vi "TraverseControl.vi"(0 "Mode":T1=enum."Read traverse position", 1 "Route Checking?":bool, 3 "Traverse Name":string, 5 "Coordinate rotation (deg)":dbl format="%.2f", 11 "Position input XYZ":dbl[](array[numeric])=[0.0, 0.0, 0.0] format="%.2f", 13 "Speed Factor":dbl=1.0 min=0.1 max=5.0 format="%.2f", 14 "Backlash Compensation?":bool=TRUE) -> (4 "Position Output XYZ":dbl[](array[numeric]) format="%.2f", 15 "Error String":string)   [LabVIEW 2010]
uses:
  Anemometry/Anemometry Sub Vis/Gen Trav/Trav_mode.ctl
  ~subVIs/GenericDriveCommand.ctl
  ADAM Client/Sub VIs/ADAM Controls/Update_scan_value.ctl
  Anemometry/Anemometry Sub Vis/Globals/Trav_pos_global.vi
  Anemometry/Anemometry Sub Vis/Globals/Preference_global.vi
  ~subVIs/DriveConfigGlobal.vi
  Anemometry/Anemometry Sub Vis/Gen Trav/Route mapping/Route_mapping_global.vi
panel:
  out "Server copy Location":path
  out "Position Steps":dbl[][](array[numeric]) format="%.2f"
  out "Log File":path
  out "Achieved Pos In Eng units of all channels":dbl[](array[numeric]) format="%.2f"
  out "Pulses Positon all channels":dbl[](array[numeric])
  out "Counters Reset?":bool
  # "X                Y                   Z"
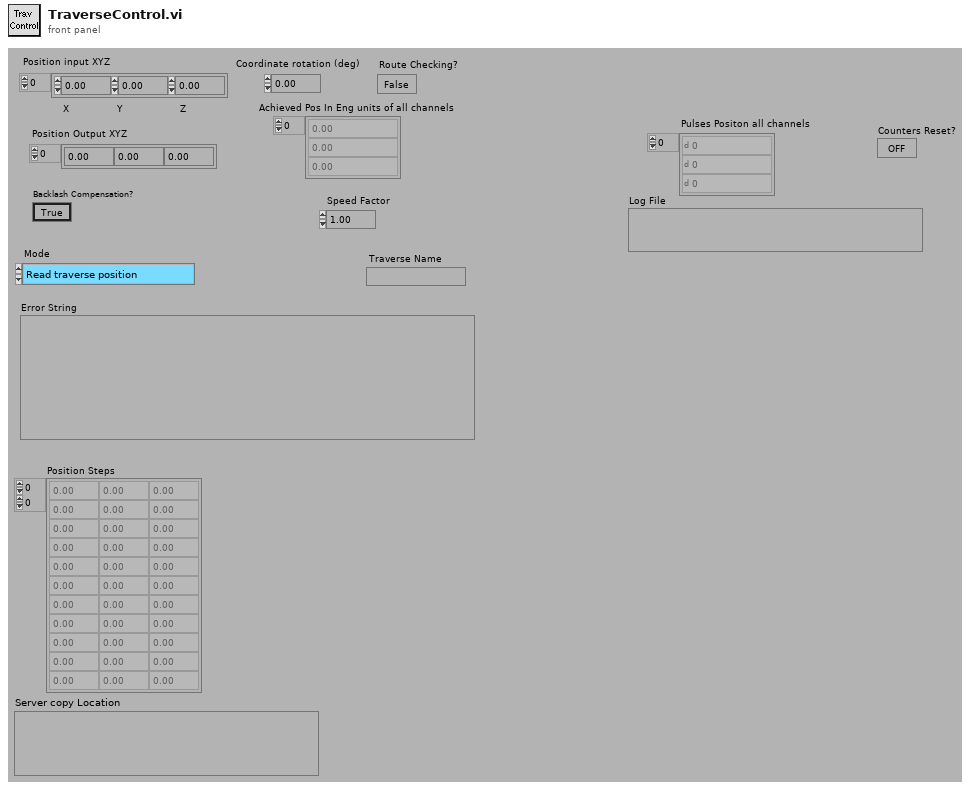
[diagram p1: front panel]
types:
  T1 = typedef "Trav_mode.ctl" = enum16{"Move traverse", "Read traverse position", "Teach Position"}
  T2 = typedef "Tunnel_Coordinates.ctl" = enum16{"Work in Tunnel Coordinates", "Work in Model Coordinates"}
  T3 = typedef "GenericDriveCommand.ctl" = string
  T4 = enum16{"To Traverse Coordinates", "To User Coordinates"}
  T5 = typedef "Update_scan_value.ctl" = cluster{"Channel Name":string, "New Value":dbl}
  T6 = typedef "AxisConfigCluster.ctl" = cluster{"Channel Properties":T7, "Static Drive Configuration":T8}
  T7 = typedef "DriveProperties.ctl" = cluster{"Channel Name":string, "Vel. Default":dbl, "Acc. Default":dbl, "Vel. Max":dbl, "Vel. Min":dbl, "Acc. Max":dbl, "Acc. Min":dbl, "Pulses/unit":dbl, "Address":u8, "Pulse Offset":i32, "Pos Tolerance":dbl, "Pulses/rev":dbl, "Backlash/Eng units":dbl, "Current Pos":dbl, "Ch Status":enum16{"Active", "Offline", "Simulate"}, "Port Name":string, "Axis Transform mode":string, "Metadata Ch Name":string, "Type":string}
  T8 = typedef "DriveStaticConfig.ctl" = cluster{"Correction Gain % (CG)":u16, "Dead Band (DB)":i32, "Dead Band Window (DW)":i32, "Encoder Resolution (ER)":i32, "Step Mode  (FSB)":u16, "Position Maintenance (FSC)":u16, "Stop on Stall (FSD)":u16, "Activate OP1 on stall (FSE)":u16, "Stop on Trigger 3 (FSF)":u16, "OP2 in Deadband (FSG)":u16, "Stall Detect (FSH)":u16, "Limit Disable (LD)":u16, "Motor Resolution (MR)":enum16{"200", "400", "1000", "2000", "4000", "5000", "10000", "12800", "18000", "20000", "21600", "25000", "25400", "25600", "36000", "50000", "278528", "425984", "507904", "614400", "655360", "819200", "1024000"}, "Limit Switch Sense (OSA)":u16, "Home Position (OSB)":u16, "Home Switch Sense (OSC)":u16, "Encoder Z for Home (OSD)":u16, "Reference edge of Home (OSH)":u16, "RS232 Echo Control (SSA)":u16, "Buffer at Limit (SSG)":u16, "Buffer at Stop (SSH)":u16, "Indexer Mode  (FSA)":u16, "Type":string, "ConfigString":string, "De Power Motor":enum16{"TRUE", "FALSE"}}
  T9 = typedef "Box_size.ctl" = cluster{"Max":dbl, "Min":dbl}[]
  T10 = typedef "Exclude_cluster.ctl" = cluster{"Sizes":T9, "Name":string, "Exclude Type":T11}
  T11 = typedef "Exclusion_type.ctl" = enum16{"Exclude completely", "Allow only vertical moves"}
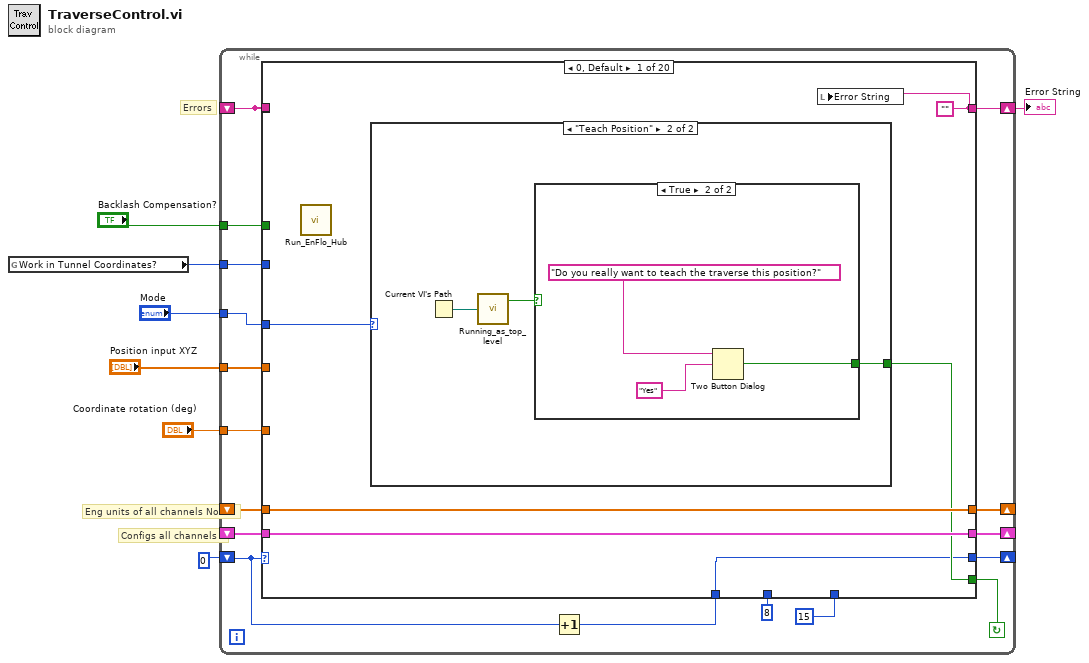
[diagram p0: block diagram]
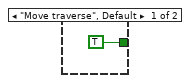
[diagram p2: hidden frame]
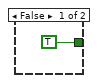
[diagram p3: hidden frame]
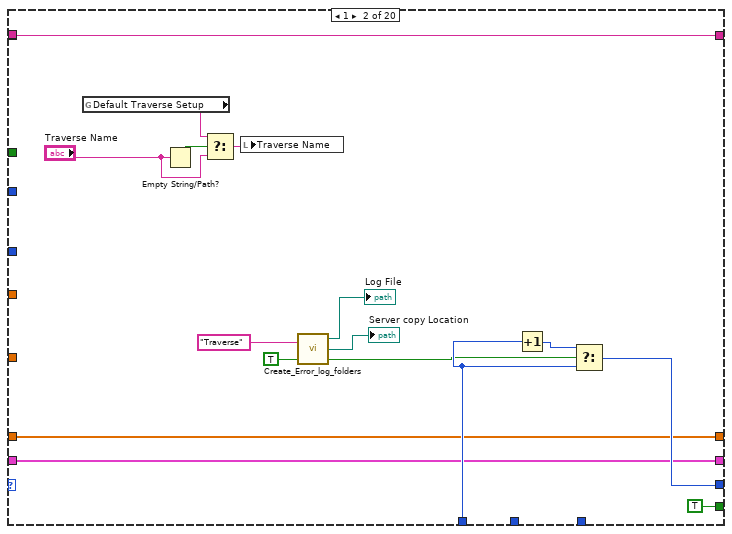
[diagram p4: hidden frame]
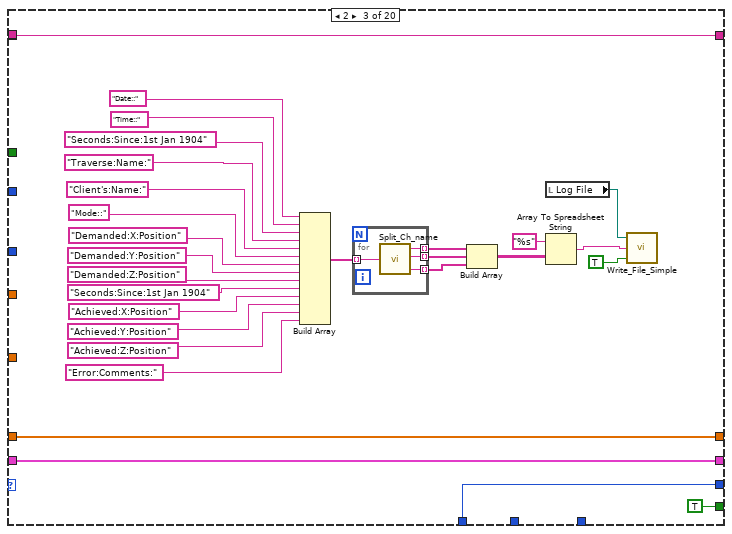
[diagram p5: hidden frame]
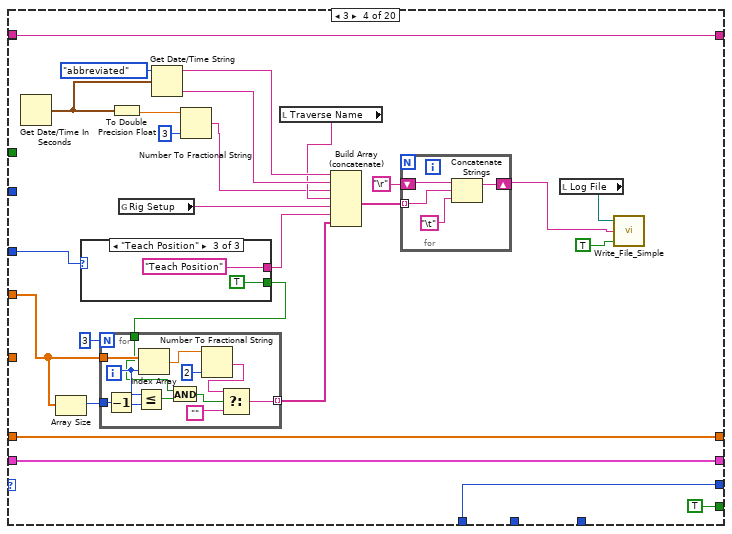
[diagram p6: hidden frame]
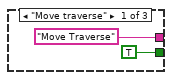
[diagram p7: hidden frame]
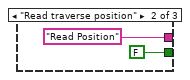
[diagram p8: hidden frame]
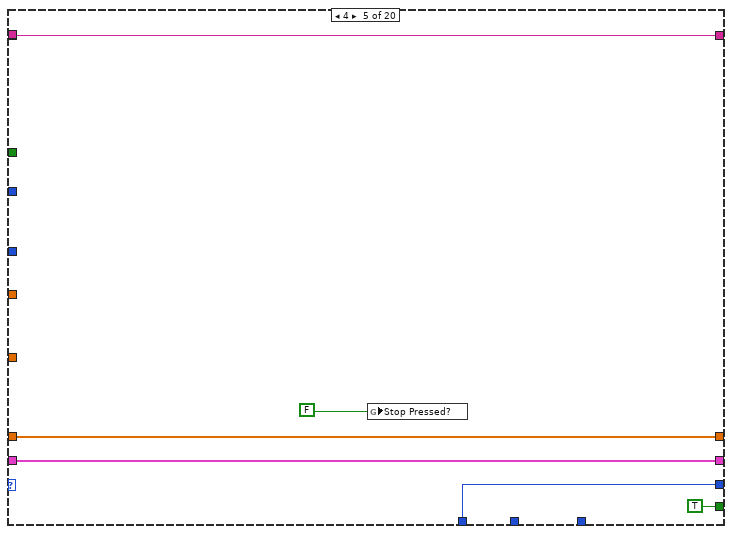
[diagram p9: hidden frame]
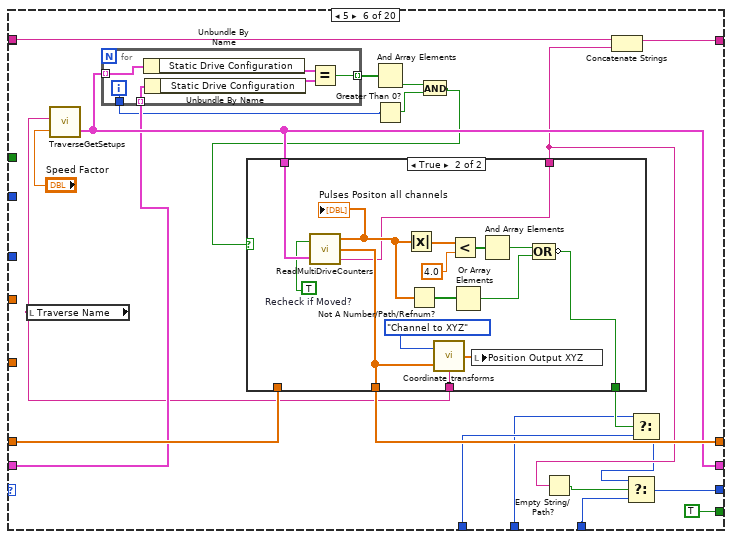
[diagram p10: hidden frame]
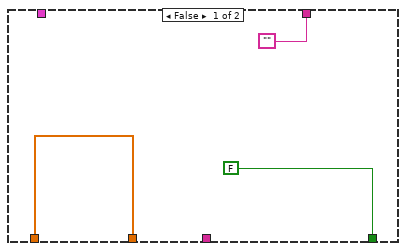
[diagram p11: hidden frame]
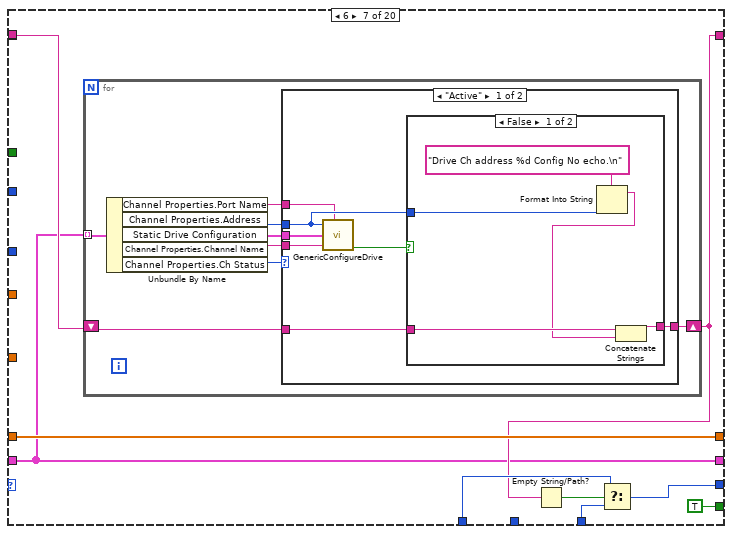
[diagram p12: hidden frame]
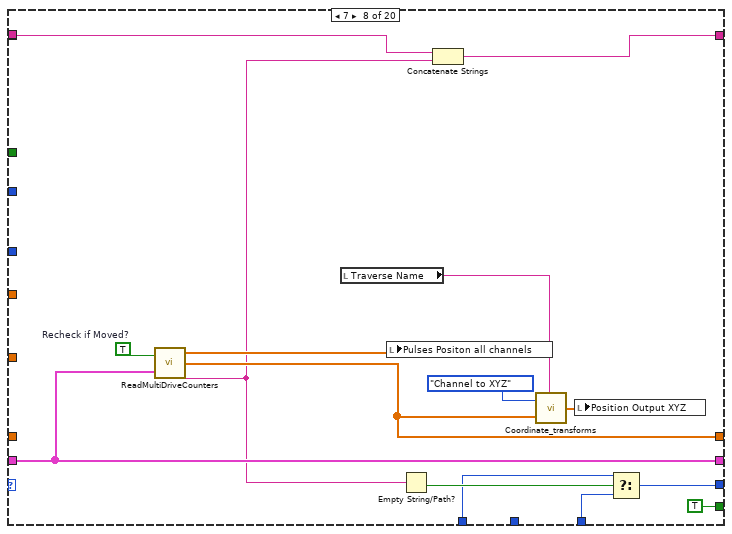
[diagram p15: hidden frame]
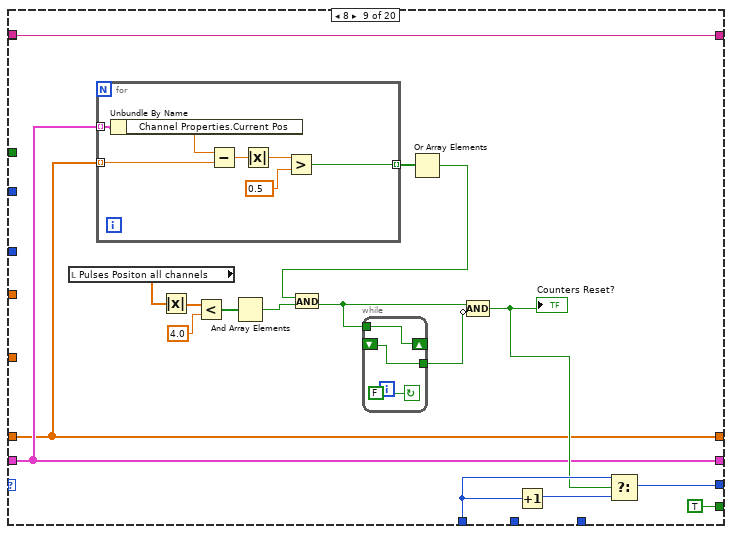
[diagram p16: hidden frame]
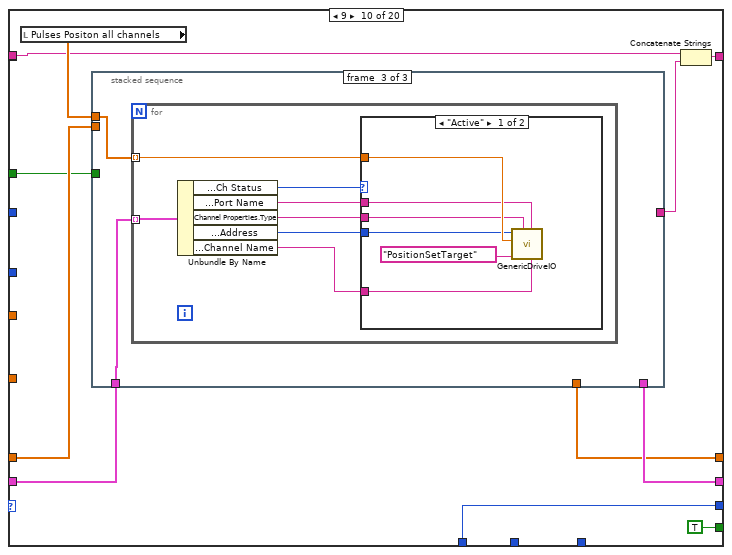
[diagram p17: hidden frame]
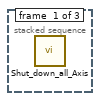
[diagram p18: hidden frame]
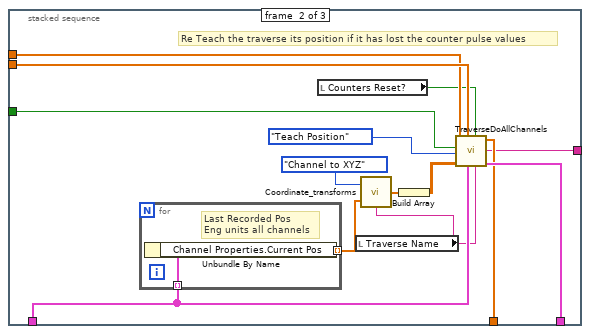
[diagram p19: hidden frame]
diagram:
  # "Errors"
  # "Eng units of all channels Now"
  # "Configs all channels"
  n1 = global read "Trav_pos_global.vi" "Work in Tunnel Coordinates?"() -> (w1:T2)
  n2 = while {
    tunnel: "Backlash Compensation?" -> [w10]
    tunnel: "Position input XYZ" -> [w14]
    shift-left: _ -> [w11]
    shift-right: [w15] -> w5
    shift-left: _ -> [w16]
    shift-right: [w17] -> _
    shift-left: _ -> [w18]
    shift-right: [w19] -> _
    shift-left: 0 -> [w22]
    shift-right: [w20] -> _
    tunnel: "Mode" -> [w24]
    tunnel: "Coordinate rotation (deg)" -> [w9]
    tunnel: w1 -> [w8]
    stop <- w23 continue-if-true
    n3 = Increment(x=w22) -> (x+1=w21:i32)
    n4 = case shown="0, Default" w22 {
      tunnel: w24 -> [w30 _ _ w105 _ _ _ _ _ _ w309 _ w373 w380 _ _ _ w457 _ w513]
      tunnel: [w27 TRUE ("T button?") TRUE ("T button?") TRUE ("T button?") TRUE TRUE ("T button?") TRUE ("T button?") TRUE ("T button?") TRUE TRUE TRUE ("T button?") TRUE ("T button?") TRUE TRUE TRUE ("T button?") TRUE ("T button?") TRUE ("T button?") w459 TRUE FALSE] -> w23
      tunnel: w21 -> [w26 w53 w62 w110 w135 w159 w192 w220 w245 w261 w308 w342 w364 w382 w409 w423 w452 w456 w491 w520]
      tunnel: [w26 w51 w62 w110 w135 w142 w191 w218 w243 w261 w307 w343 w364 w381 w409 w421 w452 w455 w491 w520] -> w20
      tunnel: [w28 w48 w64 w112 w137 w157 w187 w232 w239 w270 w305 w345 w357 w379 w411 w435 w454 w462 w489 w518] -> w19
      tunnel: w18 -> [w28 w48 w64 w112 w137 w156 w187 w232 w239 w269 w305 w345 w371 w379 w411 w435 w454 w462 w489 w518]
      tunnel: [w29 w49 w63 w111 w138 w162 w195 w227 w238 w266 w304 w329 w365 w385 w410 w434 w453 w463 w492 w521] -> w17
      tunnel: w16 -> [w29 w49 w63 w111 w138 w161 w195 _ w238 w267 w304 w329 w360 w385 w410 w434 w453 w463 w492 w521]
      tunnel: [w25 w47 w60 w102 w139 w147 w188 w223 w242 w263 w310 w334 w367 w383 w407 w425 w450 w458 w485 w514] -> w15
      tunnel: w11 -> [_ w47 w60 w102 w139 w148 w189 w224 w242 w265 w310 _ w368 w383 w407 w425 w450 w461 w487 w516]
      tunnel: w14 -> [_ _ _ w99 _ _ _ _ _ _ w303 w331 _ _ _ _ _ _ w483 _]
      tunnel: 15 ("f") -> [_ _ _ _ _ w143 w190 w219 _ _ _ w336 _ _ _ _ _ _ _ _]
      tunnel: 8 ("t") -> [_ _ _ _ _ w158 _ _ _ _ _ _ _ _ _ _ _ _ _ _]
      tunnel: w11 -> [_ _ _ _ _ _ _ _ _ _ _ w337 _ _ _ _ _ _ _ _]
      tunnel: w10 -> [_ _ _ _ _ _ _ _ _ w260 _ _ w359 _ _ _ _ _ _ _]
      tunnel: w9 -> [_ _ _ _ _ _ _ _ _ _ _ w325 _ _ _ _ _ _ w484 w511]
      tunnel: w8 -> [_ _ _ _ _ _ _ _ _ _ _ _ _ _ _ _ _ _ w481 w509]
      frame 0, Default {
        w25 = ""
        n5 = call "Run_EnFlo_Hub.vi"() -> ()  [unwired: 8 out]
        n6 = case shown="\"Teach Position\"" w30 {
          tunnel: [TRUE ("T button?") w32] -> w27
          frame "Move traverse", Default {
          }
          frame "Teach Position" {
            n7 = Current VI's Path() -> (path=w34:path)
            n8 = call "Running_as_top_level.vi"("Vi path name"=w34) -> ("Top Level"=w33:bool)  [unwired: 1 out]
            n9 = case shown="True" w33 {
              tunnel: [TRUE ("T button?") w36] -> w32
              frame False {
              }
              frame True {
                n10 = Two Button Dialog(message="Do you really want to teach the traverse this position?", 2:"Yes" ("T button name (\"OK\")")) -> (T button?=w36:bool)  [unwired: 1 out]
              }
            }
          }
        }
        n11 = local write "Error String"(w25) -> ()
      }
      frame 1 {
        n12 = global read "Trav_pos_global.vi" "Default Traverse Setup"() -> (w44:string)
        n13 = Empty String/Path?(string/path="Traverse Name") -> (empty?=w42:bool)
        n14 = Select(t=w44, s=w42, f="Traverse Name") -> (s? t:f=w41:string)
        n15 = local write "Traverse Name"(w41) -> ()
        n16 = call "Create_Error_log_folders.vi"("Per Day Log File?"=TRUE, "Log Filename"="Traverse" ("Input Element")) -> ("exists?"=w45:bool, "Server copy Location"=→"Server copy Location":path, "Local Log File"=→"Log File":path)  [unwired: 1 in]
        n17 = Increment(x=w53) -> (x+1=w52:i32)
        n18 = Select(t=w52, s=w45, f=w53) -> (s? t:f=w51:i32)
      }
      frame 2 {
        n19 = Build Array("Date::", "Time::", "Seconds:Since:1st Jan 1904", "Traverse:Name:", "Client's:Name:", "Mode::", "Demanded:X:Position", "Demanded:Y:Position", "Demanded:Z:Position", "Seconds:Since:1st Jan 1904", "Achieved:X:Position", "Achieved:Y:Position", "Achieved:Z:Position", "Error:Comments:") -> (w67:string[])
        n20 = for {
          tunnel: w67 -> [w86] mode=indexing
          tunnel: [w85] -> w68 mode=indexing
          tunnel: [w84] -> w69 mode=indexing
          tunnel: [w83] -> w70 mode=indexing
          n21 = call "Split_Ch_name.vi"("Ch name"=w86) -> ("Top level"=w85:string, "Middle"=w84:string, "Low level"=w83:string)
        }
        n22 = Build Array(w68, w69, w70) -> (w65:string[][])
        n23 = local read "Log File"() -> (w56:path)
        n24 = Array To Spreadsheet String(array=w65, 3:"%s" ("format string")) -> (spreadsheet string=w57:string)  [unwired: 1 out]
        n25 = call "Write_File_Simple.vi"("append to file? (new file:F)"=TRUE, "character string"=w57, "file path"=w56) -> ()  [unwired: 2 out]
      }
      frame 3 {
        n26 = Get Date/Time In Seconds() -> (seconds since 1Jan1904=w91:timestamp)
        n27 = Array Size(array=w99) -> (size(s)=w100:i32)
        n28 = case shown="\"Teach Position\"" w105 {
          tunnel: ["Move Traverse" "Read Position" "Teach Position"] -> w106
          tunnel: [TRUE FALSE TRUE] -> w96
          frame "Move traverse" {
          }
          frame "Read traverse position" {
          }
          frame "Teach Position" {
          }
        }
        n29 = for {
          N: 3 -> [_]
          tunnel: w99 -> [w124]
          tunnel: w100 -> [w121]
          tunnel: [w117] -> w97 mode=indexing
          tunnel: w96 -> [w113]
          i -> [w119]
          n30 = Decrement(x=w121) -> (x-1=w120:i32)
          n31 = Less Or Equal?(x=w119, y=w120) -> (x <= y?=w115:bool)
          n32 = Index Array(array=w124, index=w119) -> (element=w123:dbl)
          n33 = And(x=w113, y=w115) -> (x .and. y?=w114:bool)
          n34 = Number To Fractional String(number=w123, precision (6)=i16 2) -> (F-format string=w118:string)  [unwired: 2 out]
          n35 = Select(t=w118, s=w114, f="") -> (s? t:f=w117:string)
        }
        n36 = To Double Precision Float(number=w91) -> (double precision float=w90:dbl)
        n37 = global read "Preference_global.vi" "Rig Setup"() -> (w87:string)
        n38 = Get Date/Time String(date format (0)=enum16{"short", "long", "abbreviated"}."abbreviated", seconds (now)=w91) -> (date string=w108:string, time string=w107:string)  [unwired: 1 out]
        n39 = Number To Fractional String(number=w90, precision (6)=i16 3) -> (F-format string=w88:string)  [unwired: 2 out]
        n40 = local read "Traverse Name"() -> (w92:string)
        n41 = Build Array (concatenate)(w108, w107, w88, w92, w87, w106, w97) -> (w103:string[])
        n42 = for {
          shift-right: [w127] -> w93
          shift-left: "\r" -> [w128]
          tunnel: w103 -> [w126] mode=indexing
          n43 = Concatenate Strings(w128, w126, "\t") -> (w127:string)
        }
        n44 = local read "Log File"() -> (w94:path)
        n45 = call "Write_File_Simple.vi"("append to file? (new file:F)"=TRUE, "character string"=w93, "file path"=w94) -> ()  [unwired: 2 out]
      }
      frame 4 {
        n46 = global write "DriveConfigGlobal.vi" "Stop Pressed?"(FALSE) -> ()
      }
      frame 5 {
        n47 = local read "Traverse Name"() -> (w150:string)
        n48 = call "TraverseGetSetups.vi"("Speed Factor"="Speed Factor", "Traverse Name"=w150) -> ("Matched Configurations"=w157:T6[])  [unwired: 1 out]
        n49 = for {
          tunnel: w157 -> [w168] mode=indexing
          tunnel: w156 -> [w167] mode=indexing
          tunnel: [w164] -> w155 mode=indexing
          tunnel: [w163] -> w154
          i -> [w163]
          n50 = Unbundle By Name(w168) -> ("Static Drive Configuration"=w166:T8)
          n51 = Unbundle By Name(w167) -> ("Static Drive Configuration"=w165:T8)
          n52 = Equal?(x=w166, y=w165) -> (x = y?=w164:bool)
        }
        n53 = And Array Elements(Boolean array=w155) -> (logical AND=w152:bool)
        n54 = Greater Than 0?(x=w154) -> (x > 0?=w153:bool)
        n55 = And(x=w152, y=w153) -> (x .and. y?=w151:bool)
        n56 = case shown="True" w151 {
          tunnel: w157 -> [_ w186]
          tunnel: [w171 w176] -> w162
          tunnel: w161 -> [w171 _]
          tunnel: [FALSE w178] -> w160
          tunnel: w150 -> [_ w174]
          tunnel: ["" w172] -> w146
          frame False {
          }
          frame True {
            w173 = TRUE  # Recheck if Moved?
            n57 = call "ReadMultiDriveCounters.vi"("Recheck if Moved?"=w173, "Matched Configurations"=w186) -> ("Pulses"=w181:dbl[], "Eng units"=w176:dbl[], "Error String"=w172:string)
            "Pulses Positon all channels" <- w181
            n58 = Absolute Value(x=w181) -> (abs(x)=w185:dbl[])
            n59 = Not A Number/Path/Refnum?(number/path/refnum=w181) -> (NaN/Path/Refnum?=w180:bool[])
            n60 = call "Coordinate_transforms.vi"("Traverse Name"=w174, "Input"=w176, "Mode"=enum16{"XYZ to Channel", "Channel to XYZ"}."Channel to XYZ") -> ("Output"=w175:dbl[])
            n61 = Less?(x=w185, y=4.0 ("Achieved Position")) -> (x < y?=w183:bool[])
            n62 = Or Array Elements(Boolean array=w180) -> (logical OR=w179:bool)
            n63 = local write "Position Output XYZ"(w175) -> ()
            n64 = And Array Elements(Boolean array=w183) -> (logical AND=w182:bool)
            n65 = Compound Arithmetic op=OR(w182, w179) -> (invert w178:bool)
          }
        }
        n66 = Empty String/Path?(string/path=w146) -> (empty?=w145:bool)
        n67 = Concatenate Strings(w148, w146) -> (w147:string)
        n68 = Select(t=w158, s=w160, f=w159) -> (s? t:f=w144:i32)
        n69 = Select(t=w144, s=w145, f=w143) -> (s? t:f=w142:i32)
      }
      frame 6 {
        n70 = for {
          tunnel: w187 -> [w203] mode=indexing
          shift-right: [w196] -> w188
          shift-left: w189 -> [w197]
          n71 = Unbundle By Name(w203) -> ("Channel Properties.Port Name"=w198:string, "Channel Properties.Address"=w202:u8, "Static Drive Configuration"=w201:T8, "Channel Properties.Channel Name"=w200:string, "Channel Properties.Ch Status"=w199:enum16{"Active", "Offline", "Simulate"})
          n72 = case shown="\"Active\"" w199 {
            tunnel: w202 -> [w208 _]
            tunnel: w201 -> [w210 _]
            tunnel: w200 -> [w209 _]
            tunnel: w198 -> [w207 _]
            tunnel: w197 -> [w205 w217]
            tunnel: [w204 w217] -> w196
            frame "Active" {
              n73 = call "GenericConfigureDrive.vi"("Address"=w208, "Port Name"=w207, "Static Drive Configuration"=w210, "Channel Name"=w209) -> ("Good Echo"=w206:bool)  [unwired: 4 out]
              n74 = case shown="False" w206 {
                tunnel: w208 -> [w215 _]
                tunnel: w205 -> [w213 w216]
                tunnel: [w212 w216] -> w204
                frame False {
                  n75 = Format Into String(format string="Drive Ch address %d Config No echo.\n" ("Format String"), w215) -> (resulting string=w211:string)  [unwired: 2 in, 1 out]
                  n76 = Concatenate Strings(w213, w211) -> (w212:string)
                }
                frame True {
                }
              }
            }
            frame "Offline", Default {
            }
          }
        }
        n77 = Empty String/Path?(string/path=w188) -> (empty?=w193:bool)
        n78 = Select(t=w192, s=w193, f=w190) -> (s? t:f=w191:i32)
      }
      frame 7 {
        w225 = TRUE  # Recheck if Moved?
        n79 = call "ReadMultiDriveCounters.vi"("Recheck if Moved?"=w225, "Matched Configurations"=w232) -> ("Pulses"=w230:dbl[], "Eng units"=w227:dbl[], "Error String"=w221:string)
        n80 = local read "Traverse Name"() -> (w226:string)
        n81 = local write "Pulses Positon all channels"(w230) -> ()
        n82 = Empty String/Path?(string/path=w221) -> (empty?=w222:bool)
        n83 = Concatenate Strings(w224, w221) -> (w223:string)
        n84 = call "Coordinate_transforms.vi"("Traverse Name"=w226, "Input"=w227, "Mode"=enum16{"XYZ to Channel", "Channel to XYZ"}."Channel to XYZ") -> ("Output"=w228:dbl[])
        n85 = local write "Position Output XYZ"(w228) -> ()
        n86 = Select(t=w220, s=w222, f=w219) -> (s? t:f=w218:i32)
      }
      frame 8 {
        n87 = local read "Pulses Positon all channels"() -> (w233:dbl[])
        n88 = for {
          tunnel: w239 -> [w259] mode=indexing
          tunnel: w238 -> [w257] mode=indexing
          tunnel: [w253] -> w236 mode=indexing
          n89 = Unbundle By Name(w259) -> ("Channel Properties.Current Pos"=w258:dbl)
          n90 = Subtract(x=w258, y=w257) -> (x-y=w256:dbl)
          n91 = Absolute Value(x=w256) -> (abs(x)=w255:dbl)
          n92 = Greater?(x=w255, y=0.5) -> (0:w253:bool)
        }
        n93 = Absolute Value(x=w233) -> (abs(x)=w249:dbl[])
        n94 = Less?(x=w249, y=4.0 ("Achieved Position")) -> (x < y?=w247:bool[])
        n95 = And Array Elements(Boolean array=w247) -> (logical AND=w237:bool)
        n96 = Or Array Elements(Boolean array=w236) -> (logical OR=w235:bool)
        n97 = And(x=w235, y=w237) -> (x .and. y?=w234:bool)
        n98 = while {
          tunnel: [w251] -> w241
          tunnel: w234 -> [w252]
          shift-left: _ -> [w251]
          shift-right: [w252] -> _
          stop <- FALSE continue-if-true
        }
        n99 = Compound Arithmetic op=AND(w234, invert w241) -> (w240:bool)
        "Counters Reset?" <- w240
        n100 = Increment(x=w245) -> (x+1=w244:i32)
        n101 = Select(t=w245, s=w240, f=w244) -> (s? t:f=w243:i32)
      }
      frame 9 {
        n102 = local read "Pulses Positon all channels"() -> (w268:dbl[])
        n103 = stacked-sequence {
          tunnel: w268 -> [_ w276 w287]
          tunnel: [_ w284 _] -> w270
          tunnel: w267 -> [_ w283 _]
          tunnel: [_ w282 _] -> w266
          tunnel: w269 -> [_ w278 w288]
          tunnel: [_ w281 _] -> w264
          tunnel: w260 -> [_ w272 _]
          frame #0 {
            n104 = call "Shut_down_all_Axis.vi"() -> ()  [unwired: 1 out]
          }
          frame #1 {
            # "Re Teach the traverse its position if it has lost the counter pulse values"
            n105 = for {
              tunnel: [w286] -> w277 mode=indexing
              tunnel: w278 -> [w285] mode=indexing
              # "Last Recorded Pos\nEng units all channels"
              n106 = Unbundle By Name(w285) -> ("Channel Properties.Current Pos"=w286:dbl)
            }
            n107 = local read "Counters Reset?"() -> (w274:bool)
            n108 = local read "Traverse Name"() -> (w273:string)
            n109 = call "Coordinate_transforms.vi"("Traverse Name"=w273, "Input"=w277, "Mode"=enum16{"XYZ to Channel", "Channel to XYZ"}."Channel to XYZ") -> ("Output"=w279:dbl[])
            n110 = Build Array(w279) -> (w271:dbl[][])
            n111 = call "TraverseDoAllChannels.vi"("Traverse Name"=w273, "Counters Reset?"=w274, "Matched Configurations all Channels In"=w278, "Current Pos In Eng units of all channels"=w283, "Position Steps"=w271, "Mode"=Trav_mode."Teach Position", "Backlash Compensation?"=w272, "Current Pulses positions for all channels"=w276) -> ("Matched Configurations Out"=w284:T6[], "Error String"=w281:string, "Achieved Pos In Eng units of all channels"=w282:dbl[])  [unwired: 1 out]
          }
          frame #2 {
            n112 = for {
              tunnel: w288 -> [w295] mode=indexing
              tunnel: w287 -> [w294] mode=indexing
              n113 = Unbundle By Name(w295) -> ("Channel Properties.Ch Status"=w293:enum16{"Active", "Offline", "Simulate"}, "Channel Properties.Port Name"=w292:string, "Channel Properties.Type"=w291:string, "Channel Properties.Address"=w290:u8, "Channel Properties.Channel Name"=w289:string)
              n114 = case shown="\"Active\"" w293 {
                tunnel: w294 -> [w301 _]
                tunnel: w292 -> [w300 _]
                tunnel: w291 -> [w299 _]
                tunnel: w290 -> [w298 _]
                tunnel: w289 -> [w297 _]
                frame "Active" {
                  n115 = call "GenericDriveIO.vi"("GenericDriveCommand"=T3 "PositionSetTarget", "Channel Name"=w297, "Numeric Value"=w301, "Address"=w298, "Type"=w299, "Port Name"=w300) -> ()  [unwired: 1 in, 5 out]
                }
                frame "Offline", Default {
                }
              }
            }
          }
        }
        n116 = Concatenate Strings(w265, w264) -> (w263:string)
      }
      frame 10 {
        n117 = Build Array(w303) -> (w302:dbl[][])
        n118 = local write "Position Steps"(w302) -> ()
        n119 = case shown="\"Read traverse position\", Default" w309 {
          tunnel: w308 -> [w311 w318]
          tunnel: [w313 w317] -> w307
          frame "Move traverse" {
            n120 = Increment(x=w311) -> (x+1=w312:i32)
            n121 = case shown="True" "Route Checking?" {
              tunnel: [w315 w316] -> w313
              tunnel: w312 -> [w315 _]
              tunnel: w311 -> [_ w316]
              frame False {
              }
              frame True {
              }
            }
          }
          frame "Read traverse position", Default {
            n122 = Increment(x=w318) -> (x+1=w317:i32)
          }
        }
      }
      frame 11 {
        w321 = 0.1  # Reduce by
        w328 = TRUE  # Full Check
        n123 = global read "Route_mapping_global.vi" "Probe Volume"() -> (w320:T9)
        n124 = local read "Traverse Name"() -> (w330:string)
        n125 = for {
          tunnel: w320 -> [w352] mode=indexing
          tunnel: [w351] -> w319 mode=indexing
          tunnel: w321 -> [w346]
          n126 = Unbundle By Name(w352) -> ("Max"=w350:dbl, "Min"=w348:dbl)
          n127 = Subtract(x=w350, y=w346) -> (x-y=w349:dbl)
          n128 = Add(x=w346, y=w348) -> (x+y=w347:dbl)
          n129 = Bundle By Name(cluster=w352, "Max"=w349, "Min"=w347) -> (w351:cluster{"Max":dbl, "Min":dbl})
        }
        n130 = global read "Route_mapping_global.vi" "Entire Space"() -> (w322:T9)
        n131 = global read "Route_mapping_global.vi" "Exclude Array"() -> (w323:T10[])
        n132 = call "Coordinate_transforms.vi"("Traverse Name"=w330, "Input"=w329, "Mode"=enum16{"XYZ to Channel", "Channel to XYZ"}."Channel to XYZ") -> ("Output"=w332:dbl[])
        n133 = call "Coordinate_rotation.vi"("Input Position"=w332, "Coordinate rotation (deg)"=w325, "Mode"=T4."To User Coordinates") -> ("Output Position"=w339:dbl[])
        n134 = call "Coordinate_rotation.vi"("Input Position"=w331, "Coordinate rotation (deg)"=w325, "Mode"=T4."To User Coordinates") -> ("Output Position"=w338:dbl[])
        n135 = call "Check_Traverse_move.vi"("Current position"=w339, "Traverse Name"=w330, "Full Check"=w328, "New Position"=w338, "Coordinate rotation (deg)"=w325, "Probe Volume"=w319, "Entire Space"=w322, "Exclude Array"=w323) -> ("Steps"=w327:dbl[][], "Error Comments"=w324:string)  [unwired: 6 out]
        n136 = Empty String/Path?(string/path=w324) -> (empty?=w335:bool)
        n137 = for {
          tunnel: w327 -> [w355] mode=indexing
          tunnel: [w354] -> w326 mode=indexing
          tunnel: w325 -> [w353]
          n138 = call "Coordinate_rotation.vi"("Input Position"=w355, "Coordinate rotation (deg)"=w353, "Mode"=T4."To Traverse Coordinates") -> ("Output Position"=w354:dbl[])
        }
        "Position Steps" <- w326
        n139 = Select(t=w342, s=w335, f=w336) -> (s? t:f=w343:i32)
        n140 = Concatenate Strings(w337, w324) -> (w334:string)
      }
      frame 12 {
        w362 = FALSE  # Counters Reset?
        n141 = local read "Pulses Positon all channels"() -> (w372:dbl[])
        n142 = local read "Traverse Name"() -> (w361:string)
        n143 = local read "Position Steps"() -> (w358:dbl[][])
        n144 = call "TraverseDoAllChannels.vi"("Traverse Name"=w361, "Counters Reset?"=w362, "Matched Configurations all Channels In"=w371, "Current Pos In Eng units of all channels"=w360, "Position Steps"=w358, "Mode"=w373, "Backlash Compensation?"=w359, "Current Pulses positions for all channels"=w372) -> ("Matched Configurations Out"=w357:T6[], "Error String"=w366:string, "Achieved Pos In Eng units of all channels"=w365:dbl[])  [unwired: 1 out]
        "Achieved Pos In Eng units of all channels" <- w365
        n145 = call "Coordinate_transforms.vi"("Traverse Name"=w361, "Input"=w365, "Mode"=enum16{"XYZ to Channel", "Channel to XYZ"}."Channel to XYZ") -> ("Output"=→"Position Output XYZ":dbl[])
        n146 = Concatenate Strings(w368, w366) -> (w367:string)
      }
      frame 13 {
        n147 = local read "Position Output XYZ"() -> (w377:dbl[])
        n148 = case shown="\"Teach Position\"" w380 {
          tunnel: w377 -> [_ w405 _]
          frame "Move traverse" {
          }
          frame "Read traverse position" {
            n149 = local write "Position input XYZ"(w405) -> ()
          }
          frame "Teach Position" {
            n150 = local write "Mode"(Trav_mode."Teach Position" ("Mode")) -> ()
          }
        }
        n151 = for {
          tunnel: w379 -> [w397] mode=indexing
          tunnel: T5 {"Channel Name"="", "New Value"=0.0} ("Update Scan Value Cluster") -> [w396]
          tunnel: w377 -> [w394] mode=indexing
          shift-right: [w392] -> w375
          shift-left: T5[] [] -> [w393]
          n152 = Unbundle By Name(w397) -> ("Channel Properties.Metadata Ch Name"=w395:string, "Channel Properties.Ch Status"=w391:enum16{"Active", "Offline", "Simulate"})
          n153 = Equal?(x=w391, y=enum16{"Active", "Offline", "Simulate"}."Active" ("Channel Properties.Ch Status")) -> (x = y?=w389:bool)
          n154 = Empty String/Path?(string/path=w395) -> (empty?=w388:bool)
          n155 = Compound Arithmetic op=AND(invert w388, w389) -> (w387:bool)
          n156 = case shown="True" w387 {
            tunnel: w396 -> [_ w404]
            tunnel: w395 -> [_ w403]
            tunnel: w394 -> [_ w402]
            tunnel: w393 -> [w398 w400]
            tunnel: [w398 w399] -> w392
            frame False {
            }
            frame True {
              n157 = Bundle By Name(cluster=w404, "Channel Name"=w403, "New Value"=w402) -> (w401:T5)
              n158 = Build Array (concatenate)(w400, w401) -> (w399:T5[])
            }
          }
        }
        n159 = global write "DriveConfigGlobal.vi" "Run Emergency stop loop"(FALSE ("Run Emergency stop loop")) -> ()
        n160 = Increment(x=w382) -> (x+1=w381:i32)
        n161 = call "Update_Current_Value_client.vi"("Don't Bother with check?"=FALSE, "Update array in"=w375) -> ()
      }
      frame 14 {
      }
      frame 15 {
        n162 = local read "Position Output XYZ"() -> (w429:dbl[])
        n163 = Array Size(array=w429) -> (size(s)=w428:i32)
        n164 = Get Date/Time In Seconds() -> (seconds since 1Jan1904=w420:timestamp)
        n165 = for {
          N: 3 -> [_]
          tunnel: w429 -> [w449]
          tunnel: w428 -> [w446]
          tunnel: [w441] -> w427 mode=indexing
          i -> [w444]
          n166 = Decrement(x=w446) -> (x-1=w445:i32)
          n167 = Less Or Equal?(x=w444, y=w445) -> (x <= y?=w443:bool)
          n168 = Index Array(array=w449, index=w444) -> (element=w448:dbl)
          n169 = Number To Fractional String(number=w448, precision (6)=i16 2) -> (F-format string=w442:string)  [unwired: 2 out]
          n170 = Select(t=w442, s=w443, f="") -> (s? t:f=w441:string)
        }
        n171 = To Double Precision Float(number=w420) -> (double precision float=w413:dbl)
        n172 = Number To Fractional String(number=w413, precision (6)=i16 3) -> (F-format string=w412:string)  [unwired: 2 out]
        n173 = call "Remove_unprintable_Char.vi"("Input String"=w425) -> ("Output String"=w426:string)
        n174 = Build Array (concatenate)(w412, w427, w426) -> (w431:string[])
        n175 = local read "Route Checking?"() -> (w424:bool)
        n176 = for {
          shift-right: [w438] -> w417
          shift-left: "" -> [w439]
          tunnel: w431 -> [w437] mode=indexing
          n177 = Concatenate Strings(w439, w437, "\t") -> (w438:string)
        }
        n178 = Increment(x=w423) -> (x+1=w422:i32)
        n179 = local read "Server copy Location"() -> (w415:path)
        n180 = local read "Log File"() -> (w418:path)
        n181 = Select(t=w422, s=w424, f=w423) -> (s? t:f=w421:i32)
        n182 = call "Write_File_Simple.vi"("append to file? (new file:F)"=TRUE, "character string"=w417, "file path"=w418) -> ("file path Out"=w416:path)  [unwired: 1 out]
        n183 = call "Updated_File_Copy.vi"("Target Path"=w415, "Source Path"=w416) -> ()  [unwired: 2 out]
      }
      frame 16 {
      }
      frame 17 {
        n184 = local read "Position Output XYZ"() -> (w464:dbl[])
        n185 = local read "Counters Reset?"() -> (w465:bool)
        n186 = Index Array(array=w464, index=2) -> (element=w470:dbl)
        n187 = Index Array(array=w464, index=0) -> (element=w472:dbl)
        n188 = Index Array(array=w464, index=1) -> (element=w471:dbl)
        n189 = Format Into String(format string="X= %.2f\tY= %.2f\tZ= %.2f" ("Format String"), w472, w471, w470) -> (resulting string=w473:string)  [unwired: 2 in, 1 out]
        n190 = case shown="\"Read traverse position\"" w457 {
          tunnel: w456 -> [w477 w479]
          tunnel: [w477 w478] -> w455
          frame "Move traverse", Default {
          }
          frame "Read traverse position" {
            n191 = Increment(x=w479) -> (x+1=w478:i32)
          }
        }
        n192 = Select(t="\nThe traverse was probably powered down since the last move. Its position has now been retaught and now all should be well.", s=w465, f="") -> (s? t:f=w466:string)
        n193 = call "Write_out_serial_log.vi"("Header message"=w473) -> ()
        n194 = Concatenate Strings(w461, w466) -> (w458:string)
        n195 = Empty String/Path?(string/path=w458) -> (empty?=w460:bool)
        n196 = Not(x=w460) -> (.not. x?=w459:bool)
      }
      frame 18 {
        # "Add demanded position"
        n197 = case shown="\"Work in Model Coordinates\"" w481 {
          tunnel: w484 -> [_ w499]
          tunnel: w483 -> [w494 w498]
          tunnel: [w494 w496] -> w482
          tunnel: [" (Tunnel Coordinates)" " (Model Coordinates)"] -> w480
          frame "Work in Tunnel Coordinates" {
          }
          frame "Work in Model Coordinates" {
            n198 = call "Coordinate_rotation.vi"("Input Position"=w498, "Coordinate rotation (deg)"=w499, "Mode"=T4."To User Coordinates") -> ("Output Position"=w496:dbl[])
          }
        }
        n199 = for {
          tunnel: w489 -> [w507] mode=indexing
          shift-right: [w502] -> w486
          shift-left: "\nDem Pos " -> [w505]
          tunnel: w482 -> [w500] mode=indexing
          n200 = Unbundle By Name(w507) -> ("Channel Properties.Channel Name"=w506:string)
          n201 = call "Split_Ch_name.vi"("Ch name"=w506) -> ("Low level"=w504:string)  [unwired: 2 out]
          n202 = Format Into String(format string="%s=%.1f, " ("Format String"), w504, w500) -> (resulting string=w501:string)  [unwired: 2 in, 1 out]
          n203 = Concatenate Strings(w505, w501) -> (w502:string)
        }
        n204 = Concatenate Strings(w487, w486, w480) -> (w485:string)
      }
      frame 19 {
        # "Add Achieved Position"
        n205 = local read "Position Output XYZ"() -> (w508:dbl[])
        n206 = case shown="\"Work in Tunnel Coordinates\"" w509 {
          tunnel: w511 -> [_ w525]
          tunnel: [w522 w524] -> w510
          tunnel: w508 -> [w522 w523]
          frame "Work in Tunnel Coordinates" {
          }
          frame "Work in Model Coordinates" {
            n207 = call "Coordinate_rotation.vi"("Input Position"=w523, "Coordinate rotation (deg)"=w525, "Mode"=T4."To User Coordinates") -> ("Output Position"=w524:dbl[])
          }
        }
        n208 = for {
          tunnel: w518 -> [w537] mode=indexing
          shift-right: [w532] -> w515
          shift-left: "\nAchieved Pos " -> [w535]
          tunnel: w510 -> [w530] mode=indexing
          n209 = Unbundle By Name(w537) -> ("Channel Properties.Channel Name"=w536:string)
          n210 = call "Split_Ch_name.vi"("Ch name"=w536) -> ("Low level"=w534:string)  [unwired: 2 out]
          n211 = Format Into String(format string="%s=%.1f, " ("Format String"), w534, w530) -> (resulting string=w531:string)  [unwired: 2 in, 1 out]
          n212 = Concatenate Strings(w535, w531) -> (w532:string)
        }
        n213 = case shown="\"Move traverse\"" w513 {
          tunnel: ["When requesting a move." "When reading position." "When teaching position."] -> w512
          frame "Move traverse" {
          }
          frame "Read traverse position" {
          }
          frame "Teach Position" {
          }
        }
        n214 = Concatenate Strings(w516, w515, w512) -> (w514:string)
      }
    }
  }
  "Error String" <- w5
